vi "WriteTotalTestTime.vi"(6 "EndTime":i32, 7 "StartTime":i32, 8 "error in (no error)":errorcluster, 10 "SubItem":string, 11 "refnum out":refnum<file>) -> (0 "error out":errorcluster, 3 "refnum out 2":refnum<file>)   [LabVIEW 2012]
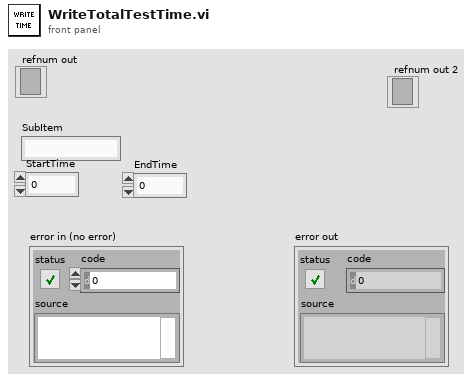
[diagram p1: front panel]
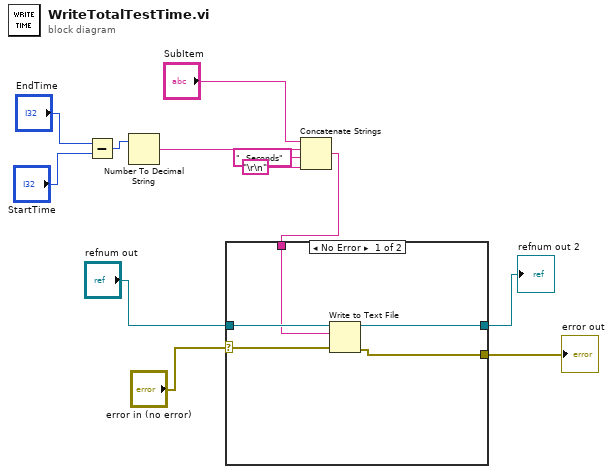
[diagram p0: block diagram]
diagram:
  n1 = Subtract(x="EndTime", y="StartTime") -> (x-y=w4:i32)
  n2 = Number To Decimal String(number=w4) -> (decimal integer string=w3:string)  [unwired: 1 in]
  n3 = Concatenate Strings("SubItem", w3, "  Seconds" ("string"), "\r\n") -> (w8:string)
  n4 = case shown="No Error" "error in (no error)" {
    selector: "error in (no error)" -> [w16 w18]
    tunnel: [w15 w18] -> w11
    tunnel: "refnum out" -> [w17 _]
    tunnel: w8 -> [w14 _]
    tunnel: [w13 _] -> w9
    frame No Error {
      n5 = Write to Text File(file (use dialog)=w17, text=w14, error in=w16) -> (refnum out=w13:refnum<file>, error out=w15:errorcluster)  [unwired: 1 in, 1 out]
    }
    frame Error {
    }
  }
  "error out" <- w11
  "refnum out 2" <- w9
